vi "FFT Max Bin Detection Loop.vi"(8 "Error":errorcluster, 11 "Source Name":refnum<k21>) -> ()   [LabVIEW 2014]
uses:
  <vilib>/Platform/TimedLoop/XDataNode/timing_clust.ctl
  <vilib>/Platform/TimedLoop/XDataNode/nitl_modes.ctl
  <vilib>/Platform/TimedLoop/XDataNode/wakeup.ctl
  <vilib>/rvi/Emulation/niFpgaSctlEmulationGetInTimedLoop.vi
  <vilib>/rvi/Emulation/niFpgaEmulationReportErrorSimple.vi
  <vilib>/rvi/Emulation/niFpgaGetClockAttributes.vi
  <vilib>/rvi/Emulation/niFpgaCriticalErrorInLSC.vi
  <vilib>/rvi/Emulation/niFpgaEmulationIsFPGAContextNoSignature.vi
  <vilib>/rvi/errors/niFpgaSetErrorForExecOnDevCompSimple.vi
  <vilib>/rvi/eio/common/nirviEmuReportErrorAndStop.vi
  <vilib>/rvi/DataTransferAndStorage/Container/Common/niFpgaContainerGetUniqueNameForEmu.vi
  <vilib>/rvi/FIFO/Fifo_Resource/nirvififoEmulationSetSize.vi
  <vilib>/rvi/FIFO/Fifo_Resource/nirviFifoEmulationQueueMgr.vi
  <instcachedir>/0/nirviFifoEmulationQueueMgr_E5CAEC123FF24DC58D834DCA3CDAA9B5.lvgen/nirviFifoEmulationQueueMgr_E5CAEC123FF24DC58D834DCA3CDAA9B5_012.vi
  <vilib>/rvi/FIFO/Fifo_Resource/nirvififoEmulationCreateLock.vi
  <vilib>/rvi/Emulation/niFpgaProcessEmulError.vi
  <vilib>/rvi/FIFO/Fifo_Resource/nirvififoEmulationObtainLock.vi
  <vilib>/rvi/FIFO/Fifo_Resource/nirvififoEmulationReleaseLock.vi
  <vilib>/rvi/occurrence/nirviWaitOnOccurrenceBase.vi
  <vilib>/rvi/errors/nirviReportUnexpectedCaseInternalError.vi
  <vilib>/rvi/errors/nirviReportUnexpectedCaseInternalError (U32).vi
  <vilib>/rvi/Memory/Memory_Emulation/niFpgaMemoryEmulationCacheClearOnFirstRun.vi
  <vilib>/rvi/Memory/Memory_Emulation/nirvimemoryEmulationManagerCache_MakeExclusive.vi
  <vilib>/rvi/Memory/Memory_Emulation/niFpgaMemoryEmulationValidateCache.vi
  <vilib>/rvi/Memory/Memory_Emulation/nirvimemoryEmulationManagerCache_InsertValue.vi
  <vilib>/Utility/error.llb/Clear Errors.vi
  <vilib>/rvi/Memory/Memory_Emulation/nirvimemoryEmulationManagerCache_ReleaseExclusive.vi
  <vilib>/rvi/Memory/Memory_Emulation/nirvimemoryEmulationManagerCache_GetValue.vi
  <vilib>/rvi/Memory/Memory_Emulation/nirvimemoryEmulationManagerCache_SetValue.vi
  <vilib>/Platform/TimedLoop/XDataNode/XDataNode.xnode
  <vilib>/rvi/DataTransferAndStorage/Container/XNode/niFpgaContainer.xnode
  <vilib>/rvi/FIFO/Fifo_Resource/nirvififoEmulationRead.vi
  <vilib>/rvi/DataTransferAndStorage/Register/Emulation/niFpgaRegisterEmulation.vi
  <vilib>/Platform/TimedLoop/XDataNode/XDNodeRunTimeDep.lvlib
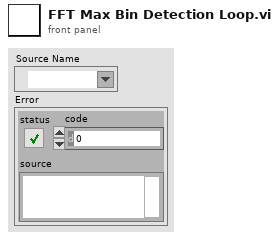
[diagram p1: front panel]
types:
  T1 = typedef "XDNodeRunTimeDep.lvlib/timing_clust.ctl" = cluster{"Expected End [f-1]":u64, "Actual End [f-1]":u64, "Finished Late? [f-1]":bool, "Expected End [i-1]":u64, "Actual End [i-1]":u64, "Finished Late? [i-1]":bool, "Expected Start [i]":u64, "Actual Start [i]":u64, "Expected Start [f]":u64, "Actual Start [f]":u64, "Source Name":string, "Structure Name":string, "Period":i64, "Deadline":i64, "Offset":i64, "Start":i64, "Priority":i32, "Timeout":i32, "Mode":T2, "Wakeup Reason":T3, "Error":errorcluster, "Source Type":string, "Secondary Source Type":string, "Global End Time":u64, "Global Start Time":u64, "Frame Duration":u64, "Iteration Duration":u64, "Assigned CPU":i32, "I/O Scan Engine Mode":u32}
  T2 = typedef "XDNodeRunTimeDep.lvlib/nitl_modes.ctl" = enum32{"No Change", "Process missed periods, maintain original phase", "Discard missed periods, maintain original phase", "Process missed periods, ignore original phase", "Discard missed periods, ignore original phase"}
  T3 = typedef "XDNodeRunTimeDep.lvlib/wakeup.ctl" = enum32{"Normal", "Aborted", "Asynchronous wakeup", "Timing source error", "Timed loop error", "Timeout"}
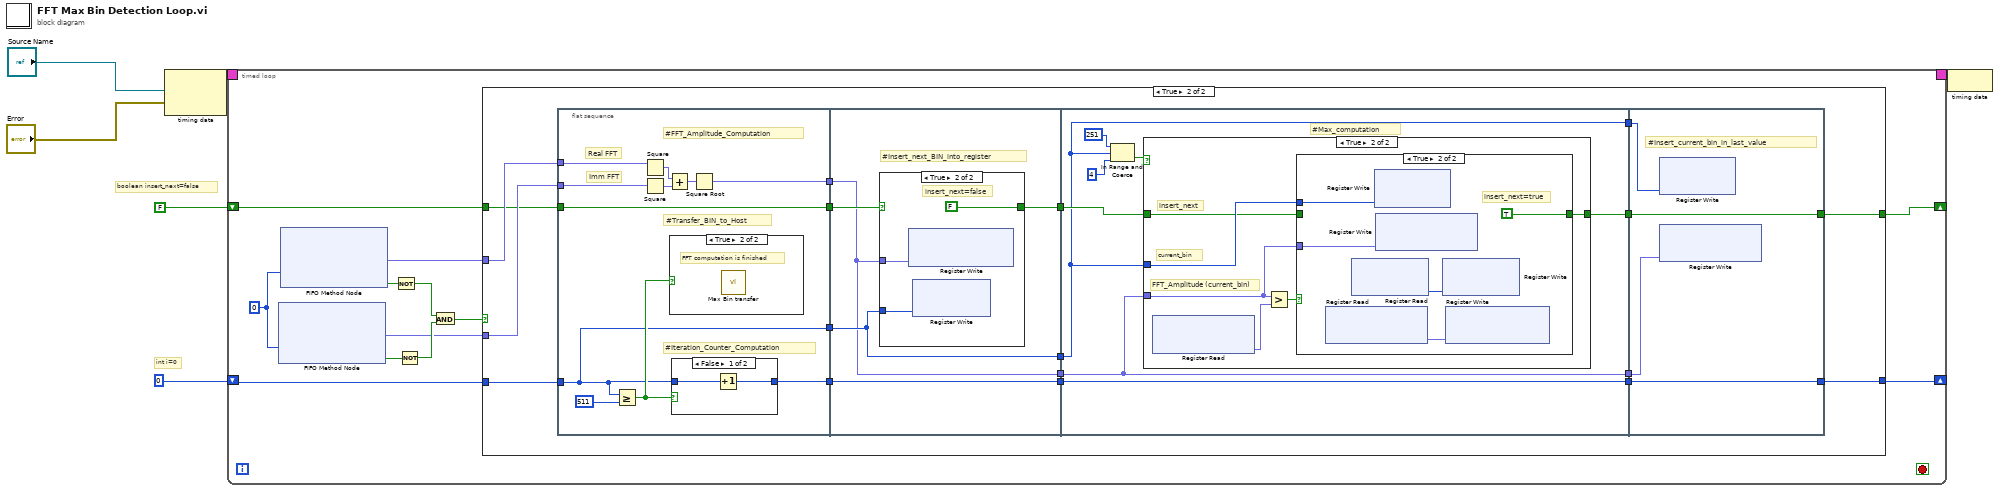
[diagram p0: block diagram]
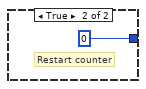
[diagram p4: hidden frame]
diagram:
  # "int i=0"
  # "boolean insert_next=false"
  n1 = node-c288("Source Name", "Error") -> (w6:T1)
  n2 = timed-loop {
    timing: w6 -> [_]
    timing-out: [_] -> w5
    shift-right: [w9] -> _
    shift-left: 0 ("Timeout") -> [w10]
    shift-right: [w7] -> _
    shift-left: FALSE -> [w8]
    stop <- _ stop-if-true
    w18 = 0 ("Timeout")
    n3 = xnode ("FIFO Method Node")("Timeout"=w18) -> ("Element"=w11:fxp<+/-,22,22>, "Timed Out?"=w16:bool)  [unwired: 1 in, 1 out]
    n4 = xnode ("FIFO Method Node")("Timeout"=w18) -> ("Element"=w12:fxp<+/-,22,22>, "Timed Out?"=w17:bool)  [unwired: 1 in, 1 out]
    n5 = Not(x=w17) -> (.not. x?=w15:bool)
    n6 = Not(x=w16) -> (.not. x?=w14:bool)
    n7 = And(x=w15, y=w14) -> (x .and. y?=w13:bool)
    n8 = case shown="True" w13 {
      tunnel: w12 -> [_ w38]
      tunnel: w11 -> [_ w37]
      tunnel: w10 -> [w20 w35]
      tunnel: [w20 w31] -> w9
      tunnel: w8 -> [w19 w28]
      tunnel: [w19 w22] -> w7
      frame False {
        # "Data are NOT ready in Target Real FFT and Target Imm FFT FIFOs"
      }
      frame True {
        n9 = flat-sequence {
          tunnel: w38 -> [w45]
          tunnel: w37 -> [w46]
          tunnel: [w44] -> w36
          tunnel: w35 -> [w40]
          tunnel: [w43] -> w34
          tunnel: [w40] -> w30
          tunnel: [w39] -> w29
          tunnel: w28 -> [w39]
          tunnel: w36 -> [w54]
          tunnel: w34 -> [w57]
          tunnel: [w57] -> w33
          tunnel: w30 -> [w55]
          tunnel: w29 -> [w56]
          tunnel: [w55] -> w27
          tunnel: [w54] -> w26
          tunnel: [w53] -> w25
          tunnel: w33 -> [w69]
          tunnel: [w69] -> w32
          tunnel: w27 -> [w64]
          tunnel: w26 -> [w63]
          tunnel: w25 -> [w65]
          tunnel: [w64] -> w24
          tunnel: [w63] -> w23
          tunnel: [w62] -> w21
          tunnel: w32 -> [w86]
          tunnel: [w86] -> w31
          tunnel: w24 -> [w85]
          tunnel: w23 -> [w84]
          tunnel: [w83] -> w22
          tunnel: w21 -> [w83]
          frame #0 {
            # "#Transfer_BIN_to_Host"
            # "#Iteration_Counter_Computation"
            # "#FFT_Amplitude_Computation"
            # "Imm FFT"
            # "Real FFT"
            n10 = Greater Or Equal?(x=w40, y=511) -> (x >= y?=w41:bool)
            n11 = Square(x=w45) -> (x^2=w49:fxp<+,43,43>)
            n12 = Square(x=w46) -> (x^2=w48:fxp<+,43,43>)
            n13 = Add(x=w49, y=w48) -> (x+y=w47:fxp<+,44,44>)
            n14 = case shown="True" w41 {
              frame False {
                # "FFT Comp is NOT finished"
              }
              frame True {
                # "FFT computation is finished"
                n15 = call "Max Bin transfer.vi"() -> ()  [unwired: 11 in, 1 out]
              }
            }
            n16 = case shown="False" w41 {
              tunnel: w40 -> [w50 _]
              tunnel: [w51 0 ("Timeout")] -> w43
              frame False {
                n17 = Increment(x=w50) -> (x+1=w51:i32)
              }
              frame True {
                # "Restart counter"
              }
            }
            n18 = Square Root(x=w47) -> (sqrt(x)=w44:fxp<+,46,22>)
          }
          frame #1 {
            # "#Insert_next_BIN_into_register"
            n19 = case shown="True" w56 {
              selector: w56 -> [w58 _]
              tunnel: [w58 FALSE] -> w53
              tunnel: w54 -> [_ w60]
              tunnel: w55 -> [_ w59]
              frame False {
              }
              frame True {
                # "insert_next=false"
                n20 = xnode "Register Write"("Data"=w60) -> ()  [unwired: 1 in, 1 out]
                n21 = xnode "Register Write"("Data"=w59) -> ()  [unwired: 1 in, 1 out]
              }
            }
          }
          frame #2 {
            # "#Max_computation"
            n22 = In Range and Coerce(upper limit=251, x=w64, lower limit=4) -> (In Range?=w66:bool)  [unwired: 1 out]
            n23 = case shown="True" w66 {
              tunnel: w63 -> [_ w74]
              tunnel: w64 -> [_ w73]
              tunnel: w65 -> [w70 w72]
              tunnel: [w70 w71] -> w62
              frame False {
                # "Current bin is NOT the maximum"
              }
              frame True {
                # "insert_next"
                # "current_bin"
                # "FFT_Amplitude (current_bin)"
                n24 = xnode "Register Read"() -> ("Data"=w76:fxp<+,46,22>)  [unwired: 1 in, 1 out]
                n25 = Greater?(x=w74, y=w76) -> (0:w75:bool)
                n26 = case shown="True" w75 {
                  tunnel: w74 -> [_ w81]
                  tunnel: w73 -> [_ w82]
                  tunnel: w72 -> [w77 _]
                  tunnel: [w77 TRUE] -> w71
                  frame False {
                  }
                  frame True {
                    # "insert_next=true"
                    n27 = xnode "Register Read"() -> ("Data"=w78:fxp<+,46,22>)  [unwired: 1 in, 1 out]
                    n28 = xnode "Register Read"() -> ("Data"=w80:i32)  [unwired: 1 in, 1 out]
                    n29 = xnode "Register Write"("Data"=w82) -> ()  [unwired: 1 in, 1 out]
                    n30 = xnode "Register Write"("Data"=w81) -> ()  [unwired: 1 in, 1 out]
                    n31 = xnode "Register Write"("Data"=w80) -> ()  [unwired: 1 in, 1 out]
                    n32 = xnode "Register Write"("Data"=w78) -> ()  [unwired: 1 in, 1 out]
                  }
                }
              }
            }
          }
          frame #3 {
            # "#Insert_current_bin_in_last_value"
            n33 = xnode "Register Write"("Data"=w85) -> ()  [unwired: 1 in, 1 out]
            n34 = xnode "Register Write"("Data"=w84) -> ()  [unwired: 1 in, 1 out]
          }
        }
      }
    }
  }
  n35 = node-c288(w5) -> ()
